vi "Real time.vi"() -> ()   [LabVIEW 2012]
uses:
  <vilib>/FPGAPlugInAG/sbRIO-9606/niLvFpga_Open_sbRIO-9606.vi
  <vilib>/rvi/interface/common/dynamic/niFpgaDynamicAddResources.vi
  <vilib>/Utility/error.llb/Error Cluster From Error Code.vi
  <vilib>/rvi/errors/niLvFpgaAdjustHostInterfaceError.vi
  <vilib>/FPGAPlugInAG/Dynamic/niLvFpga_Close_Dynamic.vi
  <vilib>/rvi/interface/nirviOpenFPGA/nirviOpenFPGA.xnode
  FPGA Bitfiles/MAX31855_FPGATarget_MAX31855_SeFi+Uu2-TQ.lvbitx
  MAX31855.vi
  <vilib>/rvi/interface/nirviReadWriteControl/nirviReadWriteControl.xnode
  <vilib>/rvi/interface/nirviCloseFPGA/nirviCloseFPGA.xnode
  NiFpgaLv.dll
  <vilib>/rvi/interface/Simulation/niFpgaSimulationCallBeginRW.vi
panel:
  out "T 1":dbl(slide) scale=0.0..100.0
  out "T 7":dbl(slide) scale=0.0..100.0
  out "T 6":dbl(slide) scale=0.0..100.0
  out "T 5":dbl(slide) scale=0.0..100.0
  out "T 4":dbl(slide) scale=0.0..100.0
  out "T 3":dbl(slide) scale=0.0..100.0
  out "T 2":dbl(slide) scale=0.0..100.0
  out "T 0":dbl(slide) scale=0.0..100.0
  in  "stop 2":bool
  in  "milliseconds to wait":u32
  in  "stop":bool
  out "Waveform Graph":dbl[](graph)
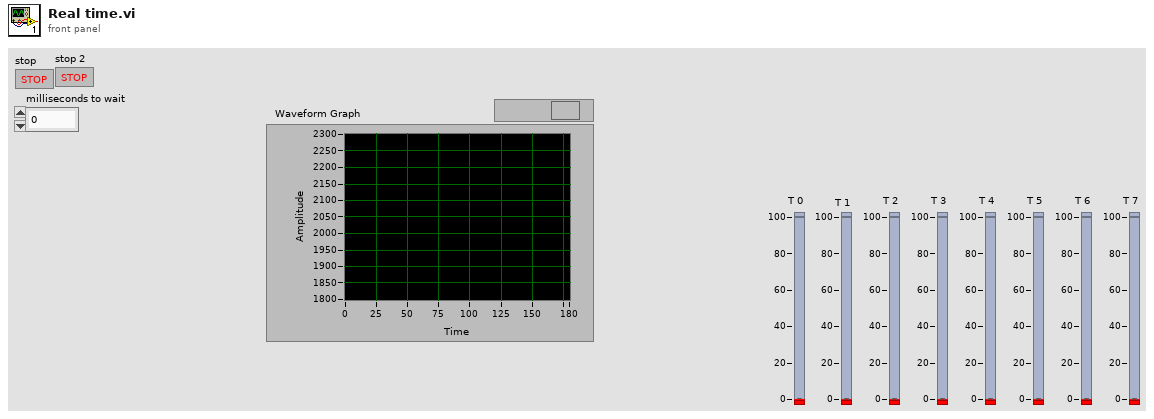
[diagram p1: front panel]
types:
  T1 = typedef "CANFrameControl.ctl" = cluster{"identifier":u32, "extended?":bool, "type":enum8{"CAN Data", "CAN Remote"}, "payload":u8[]}
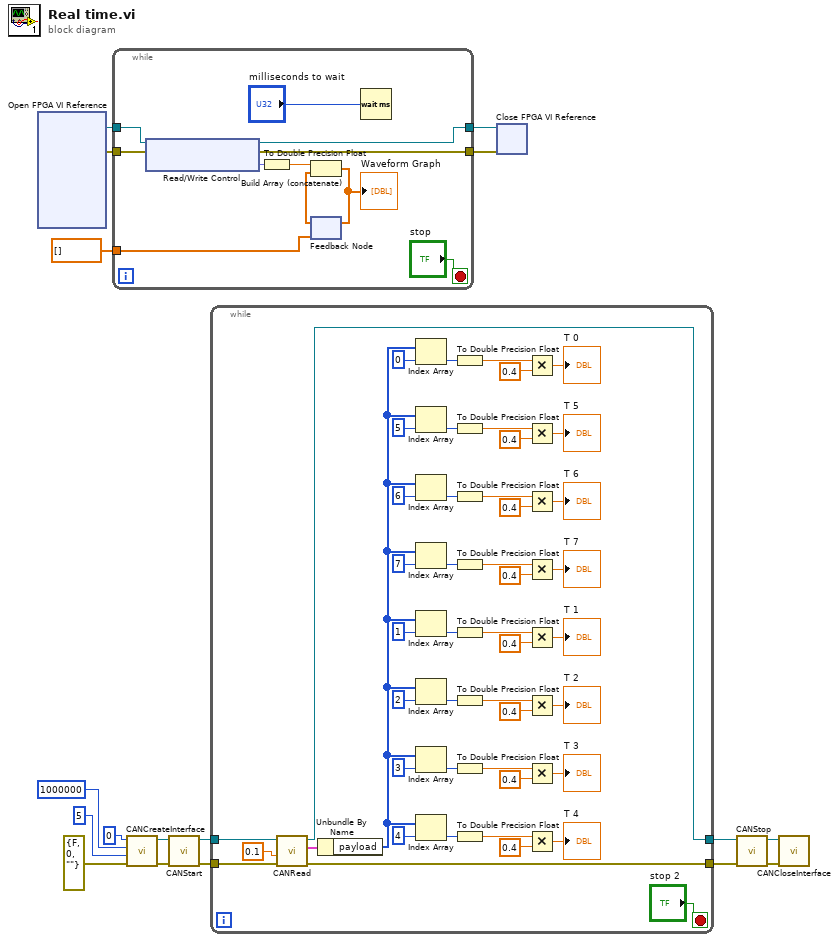
[diagram p0: block diagram]
diagram:
  n1 = xnode "Open FPGA VI Reference"() -> ("FPGA VI Reference Out"=w17:refnum<k20>, "error out"=w16:errorcluster)  [unwired: 2 in]
  n2 = while {
    tunnel: w17 -> [w28]
    tunnel: w16 -> [w27]
    tunnel: [w21] -> w15
    tunnel: [w20] -> w14
    tunnel: dbl[] [] -> [w18]
    stop <- "stop" stop-if-true
    n3 = xnode "Read/Write Control"("FPGA VI Reference In"=w28, "error in"=w27) -> ("FPGA VI Reference Out"=w21:refnum<k20>, "error out"=w20:errorcluster, "Temperatura TC 1"=w26:fxp<+,17,14>)
    n4 = To Double Precision Float(number=w26) -> (double precision float=w24:dbl)
    n5 = feedback #1(w18) -> (w23:dbl[])
    n6 = Build Array (concatenate)(w24, w23) -> (w22:dbl[])
    "Waveform Graph" <- w22
    n7 = feedback-in #1(w22) -> ()
    n8 = Wait (ms)(milliseconds to wait="milliseconds to wait") -> ()  [unwired: 1 out]
  }
  n9 = call <vilib>:"CANCreateInterface.vi"("error in (no error)"=errorcluster {"status"=FALSE, "code"=0, "source"=""}, "receive queue size"=u32 5, "baud rate"=u32 1000000, "interface index"=u32 0) -> ("error out"=w6:errorcluster, "interface object out"=w7:refnum<k20>)  [unwired: 6 in]
  n10 = call <vilib>:"CANStart.vi"("error in (no error)"=w6, "interface object in"=w7) -> ("error out"=w1:errorcluster, "interface object out"=w8:refnum<k20>)  [unwired: 8 in]
  n11 = while {
    tunnel: w8 -> [w75]
    tunnel: [w74] -> w5
    tunnel: [w73] -> w2
    tunnel: w1 -> [w71]
    stop <- "stop 2" stop-if-true
    n12 = call <vilib>:"CANRead.vi"("error in (no error)"=w71, "timeout"=0.1, "interface object in"=w75) -> ("error out"=w73:errorcluster, "CAN frame"=w70:T1, "interface object out"=w74:refnum<k20>)  [unwired: 5 in, 1 out]
    n13 = Unbundle By Name(w70) -> ("payload"=w61:u8[])
    n14 = Index Array(array=w61, index=0) -> (element=w60:u8)
    n15 = Index Array(array=w61, index=5) -> (element=w40:u8)
    n16 = Index Array(array=w61, index=6) -> (element=w41:u8)
    n17 = Index Array(array=w61, index=7) -> (element=w42:u8)
    n18 = Index Array(array=w61, index=1) -> (element=w36:u8)
    n19 = Index Array(array=w61, index=2) -> (element=w37:u8)
    n20 = Index Array(array=w61, index=3) -> (element=w38:u8)
    n21 = Index Array(array=w61, index=4) -> (element=w39:u8)
    n22 = To Double Precision Float(number=w60) -> (double precision float=w59:dbl)
    n23 = To Double Precision Float(number=w40) -> (double precision float=w48:dbl)
    n24 = To Double Precision Float(number=w41) -> (double precision float=w46:dbl)
    n25 = To Double Precision Float(number=w42) -> (double precision float=w44:dbl)
    n26 = To Double Precision Float(number=w36) -> (double precision float=w56:dbl)
    n27 = To Double Precision Float(number=w37) -> (double precision float=w54:dbl)
    n28 = To Double Precision Float(number=w38) -> (double precision float=w52:dbl)
    n29 = To Double Precision Float(number=w39) -> (double precision float=w50:dbl)
    n30 = Multiply(x=w59, y=0.4) -> (x*y=→"T 0":dbl)
    n31 = Multiply(x=w48, y=0.4) -> (x*y=→"T 5":dbl)
    n32 = Multiply(x=w46, y=0.4) -> (x*y=→"T 6":dbl)
    n33 = Multiply(x=w44, y=0.4) -> (x*y=→"T 7":dbl)
    n34 = Multiply(x=w56, y=0.4) -> (x*y=→"T 1":dbl)
    n35 = Multiply(x=w54, y=0.4) -> (x*y=→"T 2":dbl)
    n36 = Multiply(x=w52, y=0.4) -> (x*y=→"T 3":dbl)
    n37 = Multiply(x=w50, y=0.4) -> (x*y=→"T 4":dbl)
  }
  n38 = xnode "Close FPGA VI Reference"("FPGA VI Reference In"=w15, "error in"=w14) -> ()  [unwired: 1 out]
  n39 = call <vilib>:"CANStop.vi"("error in (no error)"=w2, "interface object in"=w5) -> ("error out"=w3:errorcluster, "interface object out"=w4:refnum<k20>)  [unwired: 8 in]
  n40 = call <vilib>:"CANCloseInterface.vi"("error in (no error)"=w3, "interface object in"=w4) -> ()  [unwired: 9 in, 1 out]
